vi "Qn10_Z.vi"(11 "String":string) -> (3 "Qn":dbl[](array[numeric]))   [LabVIEW 2015]
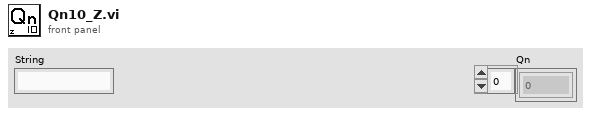
[diagram p1: front panel]
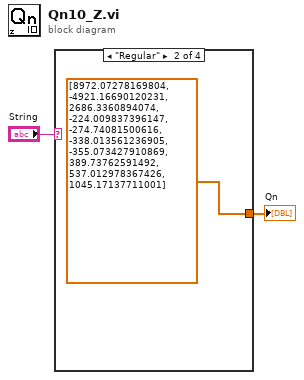
[diagram p0: block diagram]
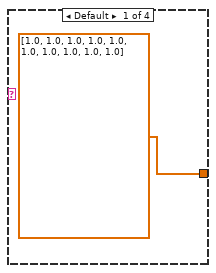
[diagram p2: hidden frame]
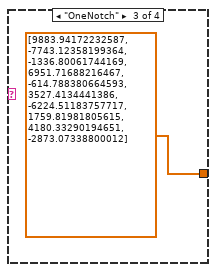
[diagram p3: hidden frame]
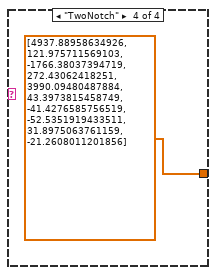
[diagram p4: hidden frame]
diagram:
  n1 = case shown="\"Regular\"" "String" {
    tunnel: [dbl[] [1.0, 1.0, 1.0, 1.0, 1.0, 1.0, 1.0, 1.0, 1.0, 1.0] ("Qn") dbl[] [8972.07278169804, -4921.16690120231, 2686.3360894074, -224.009837396147, -274.74081500616, -338.013561236905, -355.073427910869, 389.73762591492, 537.012978367426, 1045.17137711001] ("Qn") dbl[] [9883.94172232587, -7743.12358199364, -1336.80061744169, 6951.71688216467, -614.788380664593, 3527.4134441386, -6224.51183757717, 1759.81981805615, 4180.33290194651, -2873.07338800012] ("Qn") dbl[] [4937.88958634926, 121.975711569103, -1766.38037394719, 272.43062418251, 3990.09480487884, 43.3973815458749, -41.4276585756519, -52.5351919433511, 31.8975063761159, -21.2608011201856] ("Qn")] -> w2
    frame Default {
    }
    frame "Regular" {
    }
    frame "OneNotch" {
    }
    frame "TwoNotch" {
    }
  }
  "Qn" <- w2
